vi "Main Loop.vi"(8 "error in (no error)":errorcluster, 10 "Chart Notifier":refnum<notifier>, 11 "Message Queues":T1) -> (0 "error out":errorcluster)   [LabVIEW 2018, in "Flow Module.lvlib" / "Flow Module Engine.lvlib"]
uses:
  Flow Module Engine.lvlib
  Flow Message Queues.ctl
  support/Message Queue/Message Cluster.ctl
  State Cluster.ctl
  State Enum.ctl
  Feed Module/Controls/Flow Module Settings Cluster.ctl
  Mettler Toledo/Controls/Settings Cluster.ctl
  Feed Module/Controls/Flow Module Display.ctl
  <vilib>/Platform/TimedLoop/XDataNode/timing_clust.ctl
  <vilib>/Platform/TimedLoop/XDataNode/nitl_modes.ctl
  <vilib>/Platform/TimedLoop/XDataNode/wakeup.ctl
  Tag VIs/Tag FGV Operation Enum.ctl
  support/Message Queue/Enqueue Message (Single).vi
  <vilib>/Platform/TimedLoop/XDataNode/XDataNode.xnode
  support/Message Queue/Message Queue.lvlib
  <vilib>/Platform/TimedLoop/XDataNode/XDNodeRunTimeDep.lvlib
  Flow Module.lvlib
  Mettler Toledo/Mettler Toledo.lvlib
  Shared Variables/Dynamic Shared Variables.lvlib
  support/Support Library.lvlib
panel:
  out "Period (s)":dbl format="%_4g"
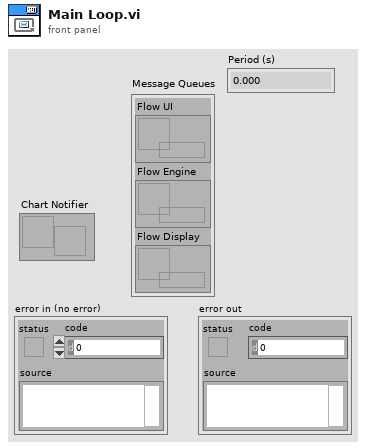
[diagram p1: front panel]
types:
  T1 = typedef "Flow Module.lvlib/Flow Message Queues.ctl" = cluster{"Flow UI":refnum<queue>, "Flow Engine":refnum<queue>, "Flow Display":refnum<queue>}
  T2 = typedef "Flow Module.lvlib/Flow Module Engine.lvlib/State Cluster.ctl" = cluster{"State":T3, "Start Time":timestamp, "Configuration":T4, "Current Time":timestamp, "First Iteration":bool, "Data":cluster{"Flow Meter Read(g/min)":dbl, "Density":dbl, "Temp (C)":dbl}, "Process Name":string, "Log Started":bool}
  T3 = typedef "Flow Module.lvlib/Flow Module Engine.lvlib/State Enum.ctl" = enum16{"Measuring", "Idle"}
  T4 = typedef "Flow Module.lvlib/Flow Module Settings Cluster.ctl" = cluster{"Cycle Period":dbl, "Bronkhorst M13":T5, "Flow Meter Type":string, "Bronkhorst M14":T5}
  T5 = typedef "Mettler Toledo.lvlib/Settings Cluster.ctl" = cluster{"VISA resource name":refnum<visa-resource-name>, "Simulated?":bool}
  T6 = typedef "XDNodeRunTimeDep.lvlib/timing_clust.ctl" = cluster{"Expected End [f-1]":u64, "Actual End [f-1]":u64, "Finished Late? [f-1]":bool, "Expected End [i-1]":u64, "Actual End [i-1]":u64, "Finished Late? [i-1]":bool, "Expected Start [i]":u64, "Actual Start [i]":u64, "Expected Start [f]":u64, "Actual Start [f]":u64, "Source Name":string, "Structure Name":string, "Period":i64, "Deadline":i64, "Offset":i64, "Start":i64, "Priority":i32, "Timeout":i32, "Mode":T7, "Wakeup Reason":T8, "Error":errorcluster, "Source Type":string, "Secondary Source Type":string, "Global End Time":u64, "Global Start Time":u64, "Frame Duration":u64, "Iteration Duration":u64, "Assigned CPU":i32, "I/O Scan Engine Mode":u32}
  T7 = typedef "XDNodeRunTimeDep.lvlib/nitl_modes.ctl" = enum32{"No Change", "Process missed periods, maintain original phase", "Discard missed periods, maintain original phase", "Process missed periods, ignore original phase", "Discard missed periods, ignore original phase"}
  T8 = typedef "XDNodeRunTimeDep.lvlib/wakeup.ctl" = enum32{"Normal", "Aborted", "Asynchronous wakeup", "Timing source error", "Timed loop error", "Timeout"}
  T9 = cluster{"enable? (F)":bool, "name":string, "alarm on":bool, "priority":u32, "ack type":enum16{"Auto", "User", "None", "Each Occurrence"}, "area":string, "description":string, "log? (T)":bool}
  T10 = typedef "Tag FGV Operation Enum.ctl" = enum16{"Init", "Set Notification Queue", "Create Tag", "Commit", "Write Tag (Numeric)", "Write Tag (Boolean)", "Read All Tags", "Read One Tag", "Delete Tag Category", "Set Alarm Parameters (Numeric)", "Set Alarm Parameters (Boolean)", "Enable All Alarms", "Disable All Alarms", "Delete All Tags", "Read Alarms", "Ack Alarm", "Read Alarm Parameters (Numeric)", "Read Alarm Parameters (Boolean)"}
  T11 = enum32{"u32BitField", "bool", "double", "string", "int8", "uint8", "int16", "uint16", "int32", "uint32", "int64", "uint64", "single", "double waveform", "int16 waveform", "array of boolean", "array of int8", "array of uint8", "array of int16", "array of uint16", "array of int32", "array of uint32", "array of int64", "array of uint64", "array of single", "array of double", "array of double waveform", "array of int16 waveform", "array of string", "variant", "timestamp", "fixed point", "custom"}
  T12 = typedef "Flow Module.lvlib/Flow Module Display.ctl" = cluster{"Flow Value":dbl, "Cycle Period":dbl, "Density":dbl, "Temp":dbl}
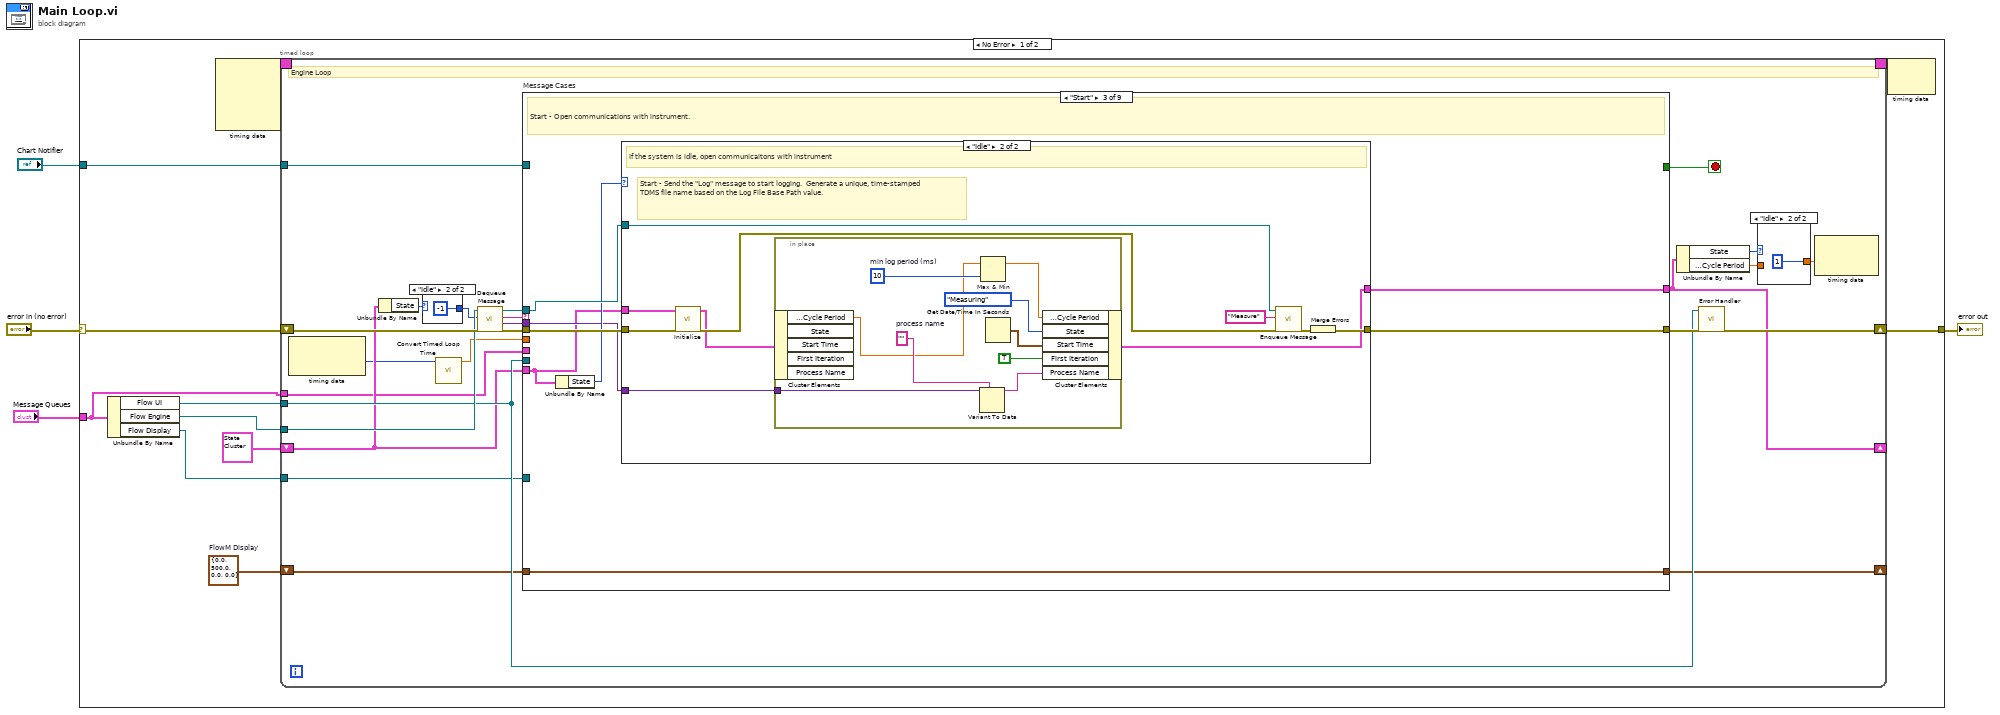
[diagram p0: block diagram]
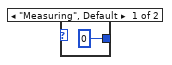
[diagram p3: hidden frame]
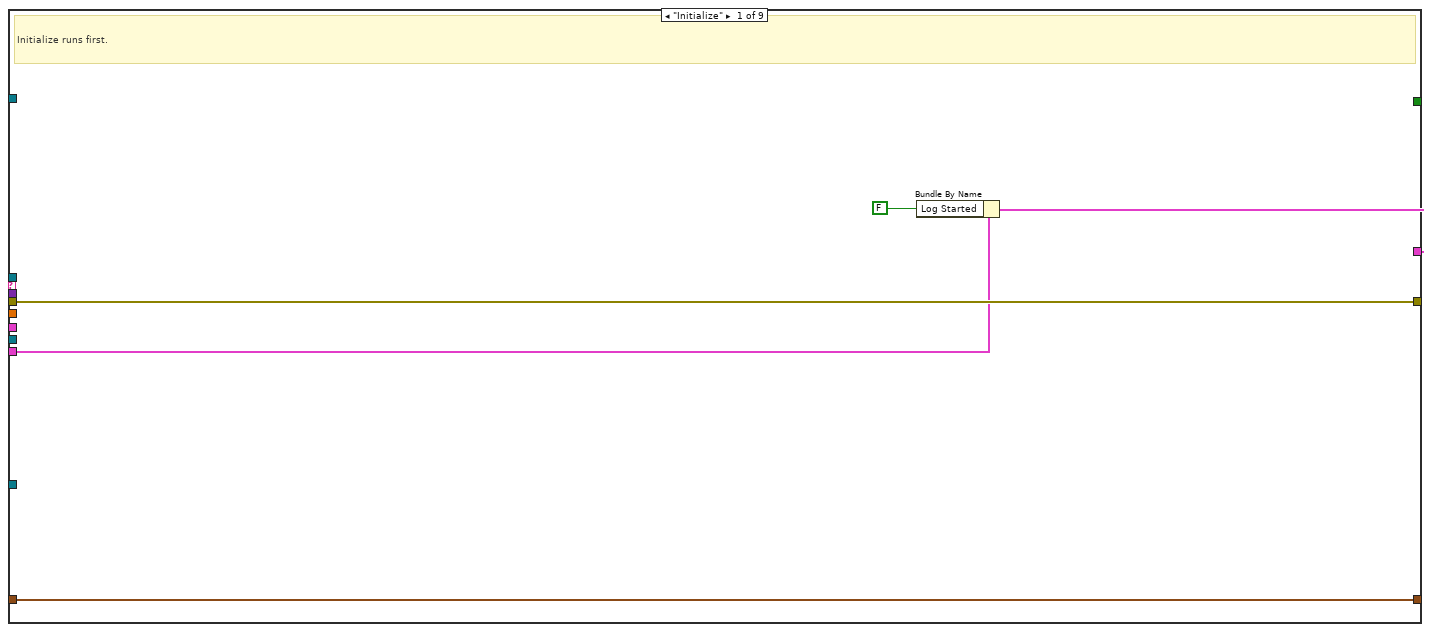
[diagram p4: hidden frame]
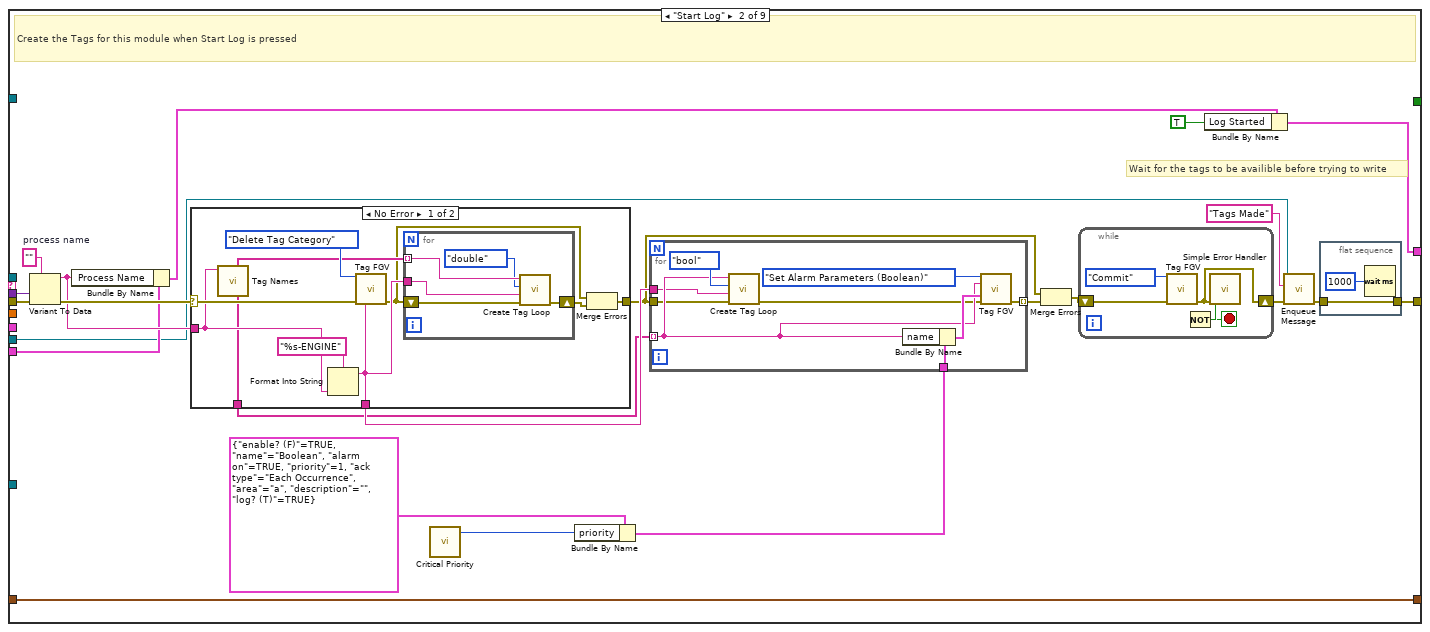
[diagram p5: hidden frame]
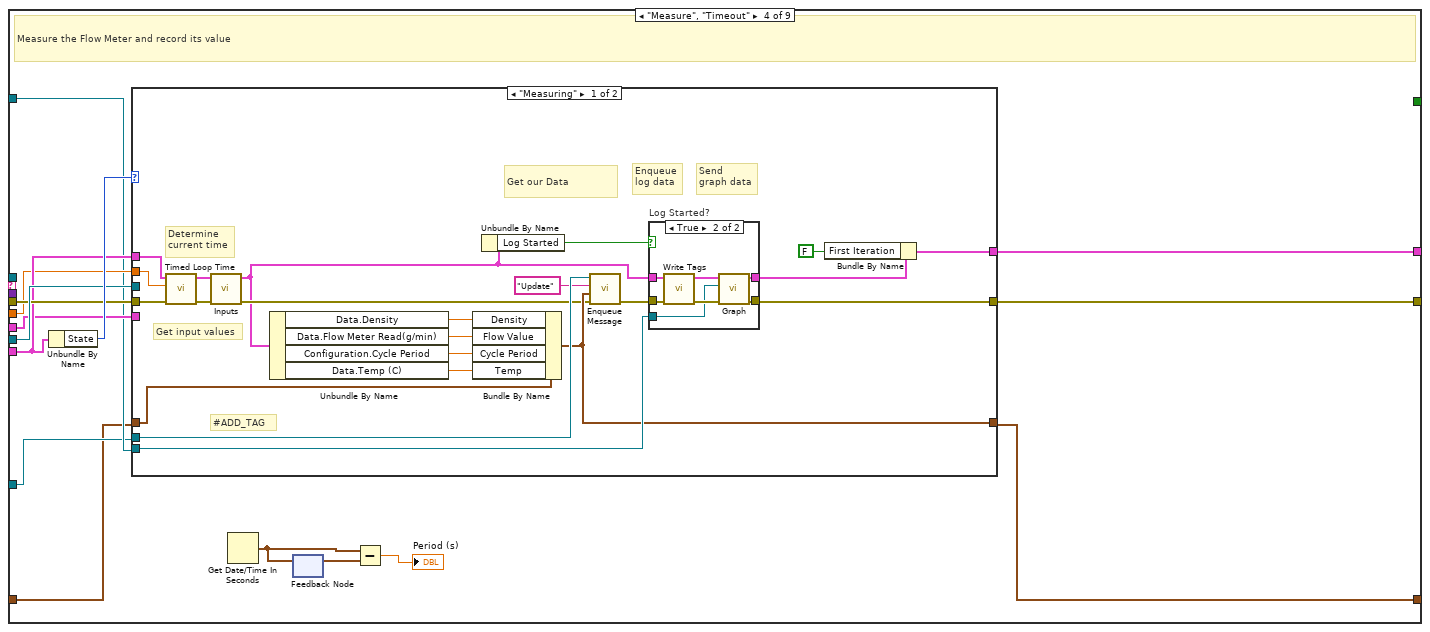
[diagram p8: hidden frame]
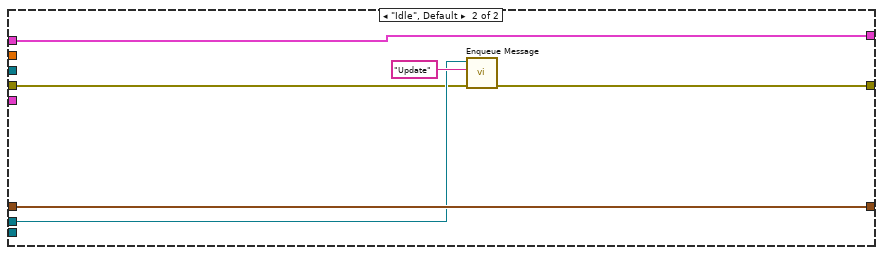
[diagram p10: hidden frame]
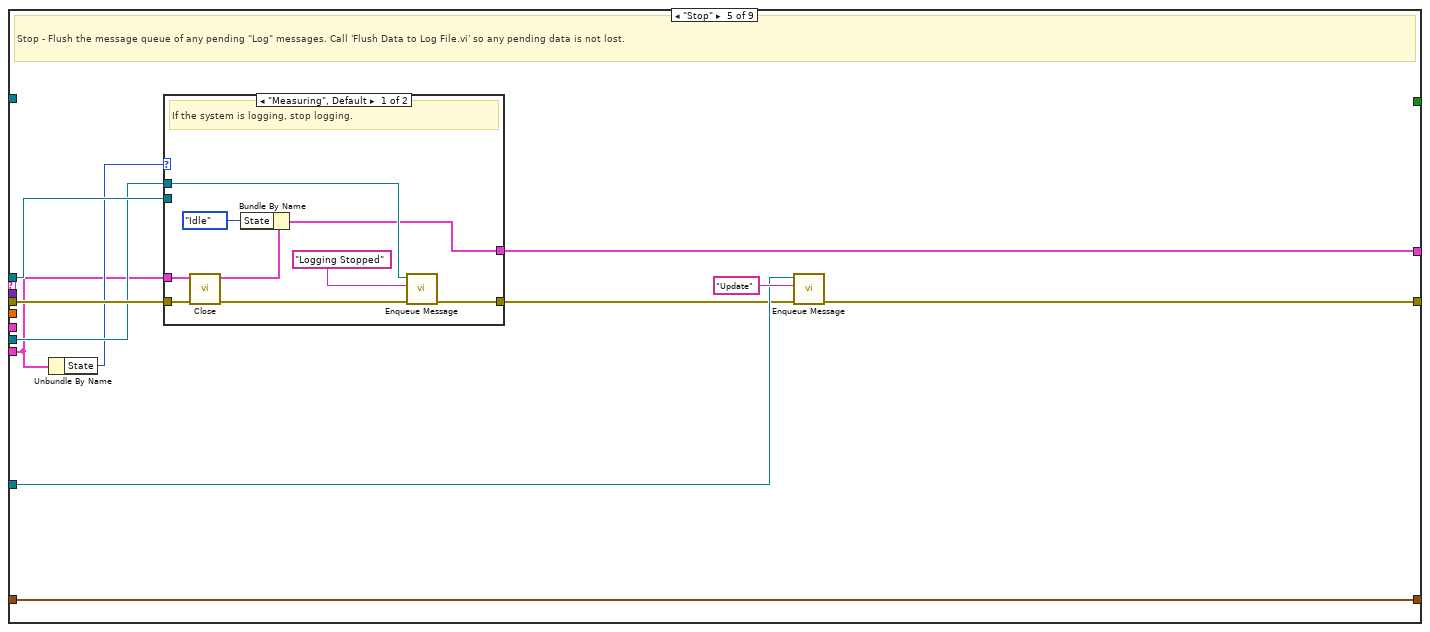
[diagram p11: hidden frame]
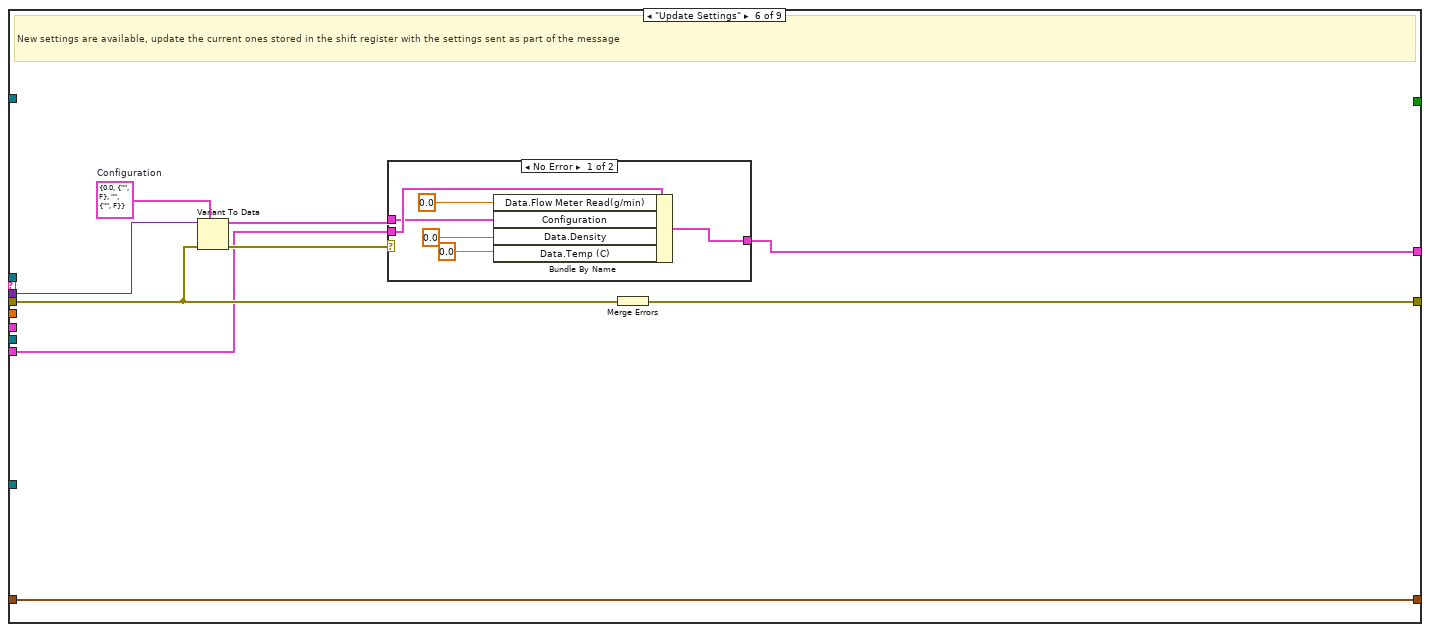
[diagram p13: hidden frame]
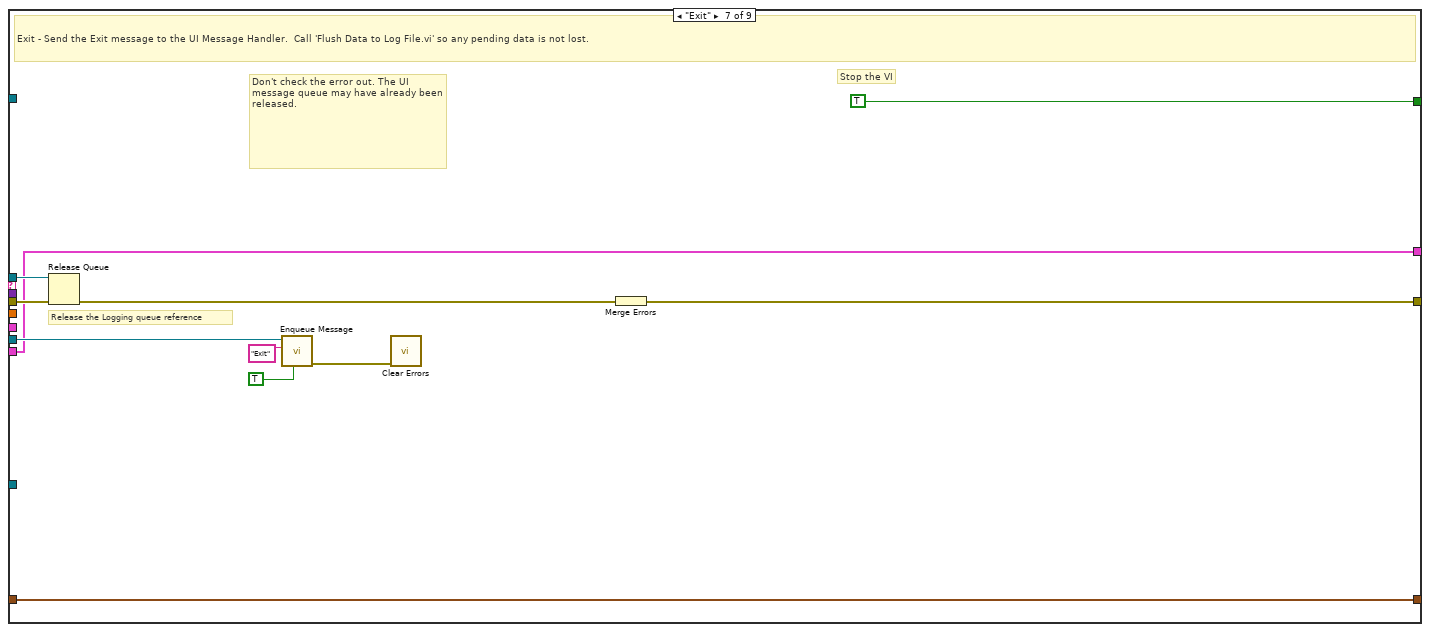
[diagram p15: hidden frame]
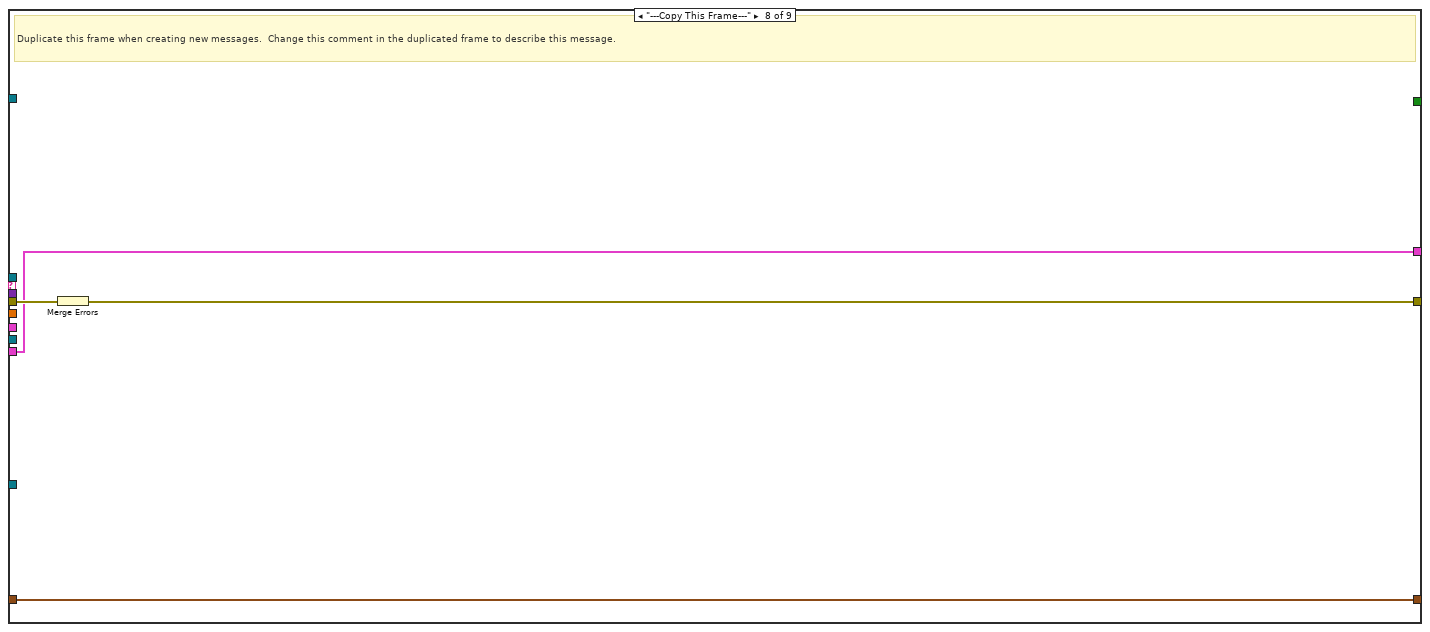
[diagram p16: hidden frame]
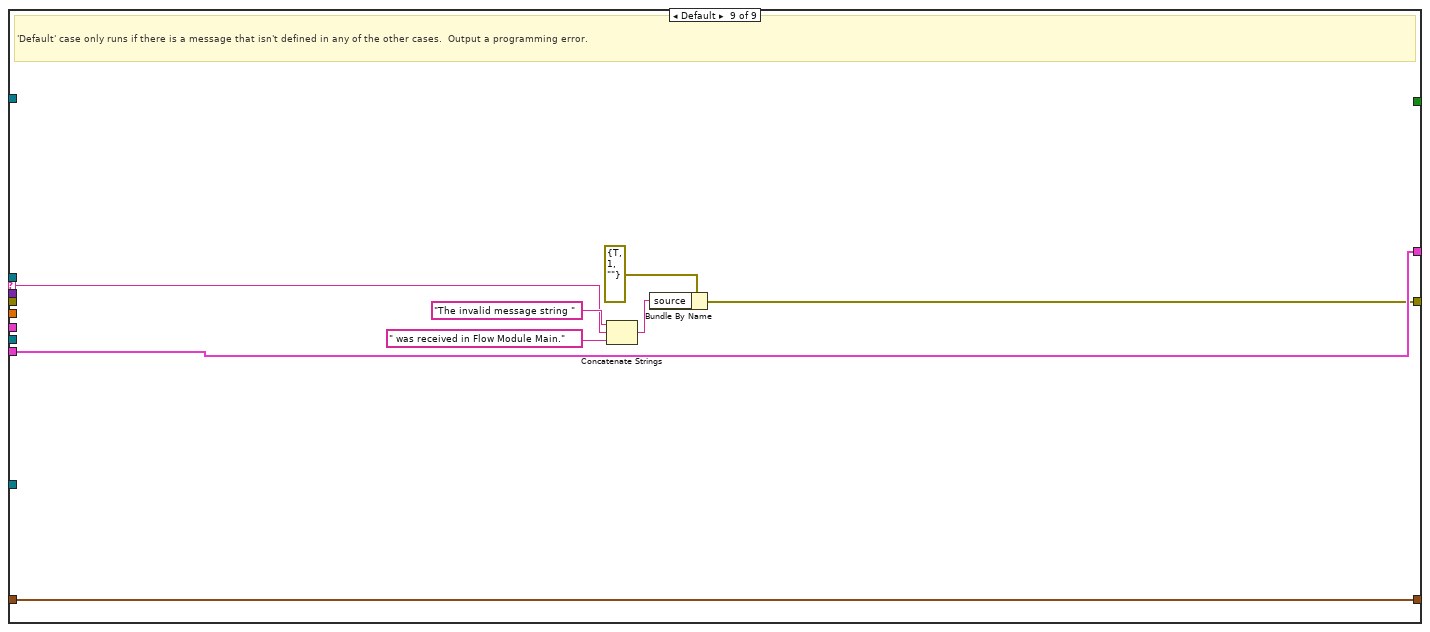
[diagram p17: hidden frame]
diagram:
  n1 = case shown="No Error" "error in (no error)" {
    selector: "error in (no error)" -> [w15 w253]
    tunnel: "Message Queues" -> [w10 _]
    tunnel: [w5 w253] -> w3
    tunnel: "Chart Notifier" -> [w8 _]
    frame No Error {
      w6 = T12 {"Flow Value"=0.0, "Cycle Period"=500.0, "Density"=0.0, "Temp"=0.0}  # FlowM Display
      n2 = Unbundle By Name(w10) -> ("Flow UI"=w14:refnum<queue>, "Flow Engine"=w9:refnum<queue>, "Flow Display"=w7:refnum<queue>)
      n3 = node-c288() -> (w12:T6)  [unwired: 4 in]
      n4 = timed-loop {
        tunnel: w9 -> [w33]
        shift-right: [w17] -> _
        shift-left: T2 {"State"=enum."Idle", "Start Time"=timestamp(0 s since 1904-01-01), "Configuration"={"Cycle Period"=0.0, "Bronkhorst M13"={"VISA resource name"="", "Simulated?"=FALSE}, "Flow Meter Type"="", "Bronkhorst M14"={"VISA resource name"="", "Simulated?"=FALSE}}, "Current Time"=timestamp(0 s since 1904-01-01), "First Iteration"=FALSE, "Data"={"Flow Meter Read(g/min)"=0.0, "Density"=0.0, "Temp (C)"=0.0}, "Process Name"="", "Log Started"=FALSE} -> [w29]
        shift-right: [w31] -> w5
        shift-left: w15 -> [w38]
        tunnel: w14 -> [w30]
        timing: w12 -> [_]
        timing-out: [_] -> w11
        tunnel: w10 -> [w21]
        tunnel: w8 -> [w20]
        tunnel: w7 -> [w19]
        shift-right: [w18] -> _
        shift-left: w6 -> [w16]
        stop <- w39 stop-if-true
        # "Engine Loop"
        n5 = node-c288() -> (w23:i64)  [unwired: 1 in, 1 out]
        n6 = Unbundle By Name(w29) -> ("State"=w28:T3)
        n7 = case shown="\"Idle\"" w28 {
          tunnel: [0 ("timeout in ms (-1)") -1 ("timeout in ms (-1)")] -> w27
          frame "Measuring", Default {
          }
          frame "Idle" {
          }
        }
        n8 = call "Convert Timed Loop Time.vi"("Actual Start [i]"=w23) -> ("ET since start (s)"=w22:dbl)  [unwired: 10 in]
        n9 = call "Dequeue Message.vi"("error in (no error)"=w38, "timeout in ms (-1)"=w27, "Message Queue"=w33) -> ("error out"=w37:errorcluster, "Message Data"=w35:variant, "Message"=w36:string, "dup Message Queue"=w34:refnum<queue>)  [unwired: 5 in]
        n10 = case "Message Cases" shown="\"Start\"" w36 {
          selector: w36 -> [_ _ _ _ _ _ _ _ w244]
          tunnel: w34 -> [_ _ w115 _ w199 _ w232 _ _]
          tunnel: w37 -> [w53 w72 w114 w149 w200 w218 w235 w242 _]
          tunnel: [w53 w56 w116 w150 w190 w220 w237 w241 w243] -> w32
          tunnel: w29 -> [w51 w71 w111 w148 w196 w216 w228 w239 w249]
          tunnel: [_ _ _ _ _ _ TRUE _ _] -> w39
          tunnel: w35 -> [_ w70 w112 _ _ w219 _ _ _]
          tunnel: w30 -> [_ w59 _ w151 w198 _ w236 _ _]
          tunnel: w22 -> [_ _ _ w147 _ _ _ _ _]
          tunnel: w21 -> [_ _ _ w146 _ _ _ _ _]
          tunnel: w20 -> [_ _ _ w142 _ _ _ _ _]
          tunnel: w19 -> [_ _ _ w141 w192 _ _ _ _]
          tunnel: w16 -> [w52 w76 w110 w140 w195 w213 w229 w240 w250]
          tunnel: [w52 w76 w110 w139 w195 w213 w229 w240 w250] -> w18
          tunnel: [w50 w62 w109 w138 w194 w212 w228 w239 w249] -> w17
          frame "Initialize" {
            # "Initialize runs first."
            n11 = Bundle By Name(cluster=w51, "Log Started"=FALSE) -> (w50:T2)
          }
          frame "Start Log" {
            w75 = ""  # process name
            # "Wait for the tags to be availible before trying to write"
            # "Create the Tags for this module when Start Log is pressed"
            n12 = Variant To Data(error in=w72, type=w75, Variant=w70) -> (data=w73:string, error out=w74:errorcluster)
            n13 = Bundle By Name(cluster=w71, "Process Name"=w73) -> (w63:T2)
            n14 = case shown="No Error" w74 {
              selector: w74 -> [w100 w108]
              tunnel: [w94 w108] -> w54
              tunnel: w73 -> [w99 _]
              tunnel: [w97 _] -> w69
              tunnel: [w96 _] -> w68
              frame No Error {
                n15 = call "Tag Names.vi"("Process Name"=w99) -> ("All Boolean Tags"=w96:string[], "All  Numeric Tags"=w98:string[])  [unwired: 8 in, 1 out]
                n16 = Format Into String(format string="%s-ENGINE", w99) -> (resulting string=w97:string)  [unwired: 2 in, 1 out]
                n17 = call "Tag FGV.vi"("Operation"=Tag_FGV_Operation_Enum."Delete Tag Category", "error in (no error)"=w100, "Tag Category"=w97) -> ("error out"=w93:errorcluster)  [unwired: 5 in, 7 out]
                n18 = for {
                  shift-right: [w103] -> w95
                  shift-left: w93 -> [w104]
                  tunnel: w97 -> [w106]
                  tunnel: w98 -> [w107] mode=indexing
                  n19 = call "Create Tag Loop.vi"("error in (no error)"=w104, "Tag Category"=w106, "data type"=T11."double", "Tag Name"=w107) -> ("error out"=w103:errorcluster)  [unwired: 7 in]
                }
                n20 = Merge Errors(w93, w95) -> (w94:errorcluster)
              }
              frame Error {
              }
            }
            n21 = call "Critical Priority.vi"() -> ("critical priority"=w65:i32)  [unwired: 11 in]
            n22 = Bundle By Name(cluster=T9 {"enable? (F)"=TRUE, "name"="Boolean", "alarm on"=TRUE, "priority"=1, "ack type"=enum."Each Occurrence", "area"="a", "description"="", "log? (T)"=TRUE} ("Boolean alarm settings"), "priority"=w65) -> (w64:T9)
            n23 = for {
              tunnel: w64 -> [w92]
              tunnel: [w91] -> w67 mode=indexing
              tunnel: w68 -> [w87] mode=indexing
              tunnel: w54 -> [w85]
              tunnel: w69 -> [w86]
              n24 = call "Create Tag Loop.vi"("error in (no error)"=w85, "Tag Category"=w86, "data type"=T11."bool", "Tag Name"=w87) -> ("error out"=w84:errorcluster)  [unwired: 7 in]
              n25 = Bundle By Name(cluster=w92, "name"=w87) -> (w90:T9)
              n26 = call "Tag FGV.vi"("Operation"=Tag_FGV_Operation_Enum."Set Alarm Parameters (Boolean)", "Tag Name"=w87, "Data"=w90, "error in (no error)"=w84) -> ("error out"=w91:errorcluster)  [unwired: 4 in, 7 out]
            }
            n27 = Merge Errors(w54, w67) -> (w58:errorcluster)
            n28 = while {
              shift-right: [w81] -> w57
              shift-left: w58 -> [w82]
              stop <- w79 stop-if-true
              n29 = call "Tag FGV.vi"("Operation"=Tag_FGV_Operation_Enum."Commit", "error in (no error)"=w82) -> ("error out"=w81:errorcluster)  [unwired: 6 in, 7 out]
              n30 = call <vilib>:"Simple Error Handler.vi"("error in (no error)"=w81) -> ("error?"=w80:bool)  [unwired: 4 in, 4 out]
              n31 = Not(x=w80) -> (.not. x?=w79:bool)
            }
            n32 = Bundle By Name(cluster=w63, "Log Started"=TRUE) -> (w62:T2)
            n33 = call-poly "Enqueue Message.vi"("error in (no error)"=w57, "Message"="Tags Made", "Message Queue"=w59) -> ("error out"=w55:errorcluster)  [unwired: 7 in, 1 out]
            n34 = flat-sequence {
              tunnel: [w77] -> w56
              tunnel: w55 -> [w77]
              frame #0 {
                n35 = Wait (ms)(milliseconds to wait=u32 1000) -> ()  [unwired: 1 out]
              }
            }
          }
          frame "Start" {
            # "Start - Open communications with instrument."
            n36 = Unbundle By Name(w111) -> ("State"=w113:T3)
            n37 = case shown="\"Idle\"" w113 {
              tunnel: [w117 w128] -> w116
              tunnel: w115 -> [_ w125]
              tunnel: w114 -> [w117 w123]
              tunnel: w111 -> [w118 w122]
              tunnel: [w118 w119] -> w109
              tunnel: w112 -> [_ w121]
              frame "Measuring", Default {
                # "The system is already running. Ignore the \"Start\" message."
              }
              frame "Idle" {
                # "Start - Send the \"Log\" message to start logging.  Generate a unique, time-stamped TDMS file name based on the Log File Base Path value."
                # "If the system is idle, open communicaitons with instrument"
                n38 = call "Initialize.vi"("error in (no error)"=w123, "State in"=w122) -> ("error out"=w124:errorcluster, "State out"=w120:T2)  [unwired: 8 in]
                n39 = in-place {
                  in-place-border: w121 -> [w135]
                  w136 = ""  # process name
                  w137 = 10  # min log period (ms)
                  n40 = in-place-cluster #1(w120) -> ("Configuration.Cycle Period"=w129:dbl)  [unwired: 4 out]
                  n41 = Variant To Data(type=w136, Variant=w135) -> (data=w130:string)  [unwired: 1 in, 1 out]
                  n42 = Max & Min(x=w129, y=w137) -> (max(x,y)=w134:dbl)  [unwired: 1 out]
                  n43 = Get Date/Time In Seconds() -> (seconds since 1Jan1904=w132:timestamp)
                  n44 = in-place-cluster #1("Configuration.Cycle Period"=w134, "State"=State_Enum."Measuring", "Start Time"=w132, "First Iteration"=TRUE, "Process Name"=w130) -> (w119:T2)
                }
                n45 = call-poly "Enqueue Message.vi"("error in (no error)"=w124, "Message"="Measure", "Message Queue"=w125) -> ("error out"=w126:errorcluster)  [unwired: 7 in, 1 out]
                n46 = Merge Errors(w126) -> (w128:errorcluster)
              }
            }
          }
          frame "Measure", "Timeout" {
            # "Measure the Flow Meter and record its value"
            n47 = Unbundle By Name(w148) -> ("State"=w152:T3)
            n48 = case shown="\"Measuring\"" w152 {
              tunnel: w149 -> [w172 w185]
              tunnel: w148 -> [w170 w188]
              tunnel: w151 -> [_ _]
              tunnel: [w174 w184] -> w150
              tunnel: [w167 w188] -> w138
              tunnel: w147 -> [w169 _]
              tunnel: w146 -> [_ _]
              tunnel: w142 -> [w165 _]
              tunnel: w141 -> [w164 w186]
              tunnel: w140 -> [w162 w189]
              tunnel: [w159 w189] -> w139
              frame "Measuring" {
                # "Get our Data"
                # "#ADD_TAG"
                # "Determine\ncurrent time"
                # "Send\ngraph data"
                # "Enqueue\nlog data"
                # "Get input values"
                n49 = call "Timed Loop Time.vi"("error in (no error)"=w172, "ET since start (s)"=w169, "State in"=w170) -> ("error out"=w173:errorcluster, "State out"=w171:T2)  [unwired: 7 in]
                n50 = call "Inputs.vi"("error in (no error)"=w173, "State in"=w171) -> ("error out"=w158:errorcluster, "State out"=w154:T2)  [unwired: 8 in]
                n51 = Unbundle By Name(w154) -> ("Data.Density"=w156:dbl, "Data.Flow Meter Read(g/min)"=w161:dbl, "Configuration.Cycle Period"=w160:dbl, "Data.Temp (C)"=w155:dbl)
                n52 = Bundle By Name(cluster=w162, "Density"=w156, "Flow Value"=w161, "Cycle Period"=w160, "Temp"=w155) -> (w159:T12)
                n53 = Unbundle By Name(w154) -> ("Log Started"=w153:bool)
                n54 = call-poly "Enqueue Message.vi"("error in (no error)"=w158, "Message Data"=w159, "Message"="Update", "Message Queue"=w164) -> ("error out"=w157:errorcluster)  [unwired: 6 in, 1 out]
                n55 = case "Log Started?" shown="True" w153 {
                  tunnel: [w176 w181] -> w174
                  tunnel: [w175 w180] -> w168
                  tunnel: w165 -> [_ w179]
                  tunnel: w157 -> [w176 w178]
                  tunnel: w154 -> [w175 w177]
                  frame False {
                  }
                  frame True {
                    n56 = call "Write Tags.vi"("error in (no error)"=w178, "State in"=w177) -> ("error out"=w182:errorcluster, "State out"=w183:T2)  [unwired: 8 in]
                    n57 = call "Graph.vi"("error in (no error)"=w182, "notifier out"=w179, "State in"=w183) -> ("error out"=w181:errorcluster, "State out"=w180:T2)  [unwired: 7 in]
                  }
                }
                n58 = Bundle By Name(cluster=w168, "First Iteration"=FALSE) -> (w167:T2)
              }
              frame "Idle", Default {
                n59 = call-poly "Enqueue Message.vi"("error in (no error)"=w185, "Message"="Update", "Message Queue"=w186) -> ("error out"=w184:errorcluster)  [unwired: 7 in, 1 out]
              }
            }
            n60 = Get Date/Time In Seconds() -> (seconds since 1Jan1904=w144:timestamp)
            n61 = feedback-in #2(w144) -> ()
            n62 = feedback #2() -> (w145:timestamp)  [unwired: 1 in]
            n63 = Subtract(x=w144, y=w145) -> (x-y=→"Period (s)":dbl)
          }
          frame "Stop" {
            # "Stop - Flush the message queue of any pending \"Log\" messages. Call 'Flush Data to Log File.vi' so any pending data is not lost."
            n64 = Unbundle By Name(w196) -> ("State"=w197:T3)
            n65 = case shown="\"Measuring\", Default" w197 {
              tunnel: [w205 w211] -> w191
              tunnel: w200 -> [w202 w211]
              tunnel: w199 -> [_ _]
              tunnel: w198 -> [w209 _]
              tunnel: w196 -> [w203 w210]
              tunnel: [w207 w210] -> w194
              frame "Measuring", Default {
                # "If the system is logging, stop logging."
                n66 = call "Close.vi"("error in (no error)"=w202, "State in"=w203) -> ("error out"=w201:errorcluster, "State out"=w204:T2)  [unwired: 8 in]
                n67 = Bundle By Name(cluster=w204, "State"=State_Enum."Idle") -> (w207:T2)
                n68 = call-poly "Enqueue Message.vi"("error in (no error)"=w201, "Message"="Logging Stopped", "Message Queue"=w209) -> ("error out"=w205:errorcluster)  [unwired: 7 in, 1 out]
              }
              frame "Idle" {
                # "The system is already idle. Ignore the \"Stop\" message."
              }
            }
            n69 = call-poly "Enqueue Message.vi"("error in (no error)"=w191, "Message"="Update", "Message Queue"=w192) -> ("error out"=w190:errorcluster)  [unwired: 7 in, 1 out]
          }
          frame "Update Settings" {
            w214 = T4 {"Cycle Period"=0.0, "Bronkhorst M13"={"VISA resource name"="", "Simulated?"=FALSE}, "Flow Meter Type"="", "Bronkhorst M14"={"VISA resource name"="", "Simulated?"=FALSE}}  # Configuration
            # "New settings are available, update the current ones stored in the shift register with the settings sent as part of the message"
            n70 = Variant To Data(error in=w218, type=w214, Variant=w219) -> (data=w215:T4, error out=w217:errorcluster)
            n71 = case shown="No Error" w217 {
              tunnel: w216 -> [w226 w227]
              tunnel: w215 -> [w225 _]
              tunnel: [w224 w227] -> w212
              frame No Error {
                n72 = Bundle By Name(cluster=w226, "Data.Flow Meter Read(g/min)"=0.0 ("Data.Scale Read(g)"), "Configuration"=w225, "Data.Density"=0.0, "Data.Temp (C)"=0.0 ("Data.Density")) -> (w224:T2)
              }
              frame Error {
              }
            }
            n73 = Merge Errors(w218) -> (w220:errorcluster)
          }
          frame "Exit" {
            # "Release the Logging queue reference"
            # "Don't check the error out. The UI message queue may have already been released."
            # "Stop the VI"
            # "Exit - Send the Exit message to the UI Message Handler.  Call 'Flush Data to Log File.vi' so any pending data is not lost."
            n74 = Release Queue(queue=w232, error in (no error)=w235) -> (error out=w231:errorcluster)  [unwired: 1 in, 2 out]
            n75 = call-poly "Enqueue Message.vi"("Priority Message? (F)"=TRUE, "Message"="Exit", "Message Queue"=w236) -> ("error out"=w230:errorcluster)  [unwired: 7 in, 1 out]
            n76 = call <vilib>:"Clear Errors.vi"("error in (no error)"=w230) -> ()  [unwired: 5 in, 2 out]
            n77 = Merge Errors(w231) -> (w237:errorcluster)
          }
          frame "---Copy This Frame---" {
            # "Duplicate this frame when creating new messages.  Change this comment in the duplicated frame to describe this message."
            n78 = Merge Errors(w242) -> (w241:errorcluster)
          }
          frame Default {
            # "'Default' case only runs if there is a message that isn't defined in any of the other cases.  Output a programming error."
            n79 = Concatenate Strings("The invalid message string " ("string"), w244, " was received in Flow Module Main." ("string")) -> (w245:string)
            n80 = Bundle By Name(cluster=errorcluster {"status"=TRUE, "code"=1, "source"=""} ("error constant"), "source"=w245) -> (w243:errorcluster)
          }
        }
        n81 = Unbundle By Name(w17) -> ("State"=w26:T3, "Configuration.Cycle Period"=w24:dbl)
        n82 = call "Error Handler.vi"("error in (no error)"=w32, "Message Queue"=w30) -> ("dup error in"=w31:errorcluster)  [unwired: 8 in, 1 out]
        n83 = case shown="\"Idle\"" w26 {
          tunnel: [w40 1] -> w25
          tunnel: w24 -> [w40 _]
          frame "Measuring" {
          }
          frame "Idle" {
          }
        }
        n84 = node-c288(w25) -> ()  [unwired: 1 in, 1 out]
      }
      n85 = node-c288(w11) -> ()  [unwired: 1 out]
    }
    frame Error {
    }
  }
  "error out" <- w3
